vi "IECMemory.contents.vi"   [LabVIEW 2014, in "IECMemory.lvlib"]
uses:
  IECMemory.lvlib
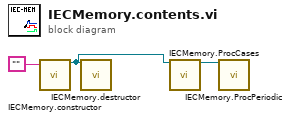
[diagram p0: block diagram]
diagram:
  n1 = call "IECMemory.constructor.vi"("name"="") -> ("i ref out"=w1:refnum<vi>)  [unwired: 16 in, 2 out]
  n2 = call "IECMemory.destructor.vi"("i ref in"=w1) -> ()  [unwired: 18 in, 1 out]
  n3 = call "IECMemory.ProcCases.vi"("i ref in"=w1) -> ("i ref out"=w2:refnum<vi>)  [unwired: 16 in, 2 out]
  n4 = call "IECMemory.ProcPeriodic.vi"("i ref in"=w2) -> ()  [unwired: 16 in, 3 out]
